vi "StopProcesses.vi"(8 "error in (no error)":errorcluster, 9 "timeout in ms (-1)":i32=-1, 11 "SMO":refnum<class "SMO.lvclass">) -> (0 "error out":errorcluster, 3 "SMO out":refnum<class "SMO.lvclass">)   [LabVIEW 2021, in "smo.lvlib" / "SMO.lvclass"]
doc: "Stops all processes in the JKI SMO.\n\n---------------------------------------------------------------\nJKI State Machine Objects™\nhttp://jki.net/state-machine-objects/\nCopyright (C) 2005-2015, JKI <info@jki.net>\nALL RIGHTS RESERVED"
uses:
  SMO.lvclass
  Typedefs/SMOState --Enum.ctl
  SMO.lvclass/SMO.ctl
  Protected/GetProtectedEvents.vi
  ReftoDVR--SMO.vi
panel:
  # "For instructions on how to use the JKI State Machine Objects, examples and video tutorials, visit:\nhttp://jki.net/state-machine-objects/\n\nJKI State Machine Objects™\nhttp://jki.net/state-machine-objects/\nCopyright (C) 2005-2015, JKI <info@jki.net>\nALL RIGHTS RESERVED"
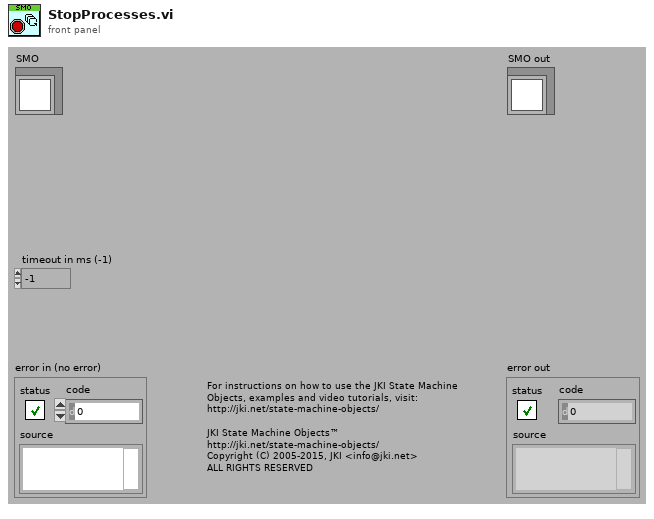
[diagram p1: front panel]
types:
  T1 = typedef "smo.lvlib/SMO.lvclass/SMOState --Enum.ctl" = enum16{"unknown", "Created", "Started", "Stopped"}
  T2 = typedef "smo.lvlib/SMO.lvclass/Process Error Notification--Cluster.ctl" = cluster{"error":errorcluster}
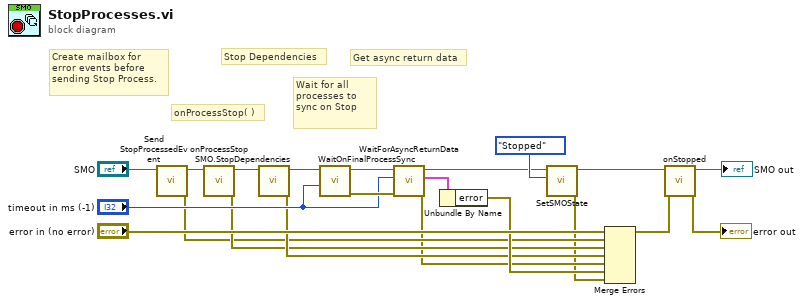
[diagram p0: block diagram]
diagram:
  # "Stop Dependencies"
  # "Get async return data"
  # "Wait for all processes to sync on Stop"
  # "onProcessStop( )"
  # "Create mailbox for\nerror events before\nsending Stop Process."
  n1 = call "Send StopProcessedEvent.vi"("SMO"="SMO") -> ("error out"=w7:errorcluster, "SMO out"=w20:refnum<class "SMO.lvclass">)  [unwired: 9 in]
  n2 = call-dynamic "onProcessStop.vi"("SMO"=w20) -> ("error out"=w8:errorcluster, "SMO out"=w12:refnum<class "SMO.lvclass">)  [unwired: 9 in]
  n3 = call "SMO.StopDependencies.vi"("SMO in"=w12) -> ("error out"=w9:errorcluster, "SMO out"=w11:refnum<class "SMO.lvclass">)  [unwired: 9 in]
  n4 = call "WaitOnFinalProcessSync.vi"("timeout in ms (-1)"="timeout in ms (-1)", "SMO"=w11) -> ("error out"=w14:errorcluster, "SMO out"=w15:refnum<class "SMO.lvclass">)  [unwired: 8 in]
  n5 = call "WaitForAsyncReturnData.vi"("error in (no error)"=w14, "timeout in ms (-1)"="timeout in ms (-1)", "SMO"=w15) -> ("error out"=w6:errorcluster, "Process Notification"=w16:T2, "SMO out"=w5:refnum<class "SMO.lvclass">)  [unwired: 6 in]
  n6 = Unbundle By Name(w16) -> ("error"=w10:errorcluster)
  n7 = call "SetSMOState.vi"("SMO State"=SMOState_--Enum."Stopped" ("event data"), "SMO in"=w5) -> ("error out"=w3:errorcluster, "SMO out"=w4:refnum<class "SMO.lvclass">)  [unwired: 8 in]
  n8 = Merge Errors("error in (no error)", w7, w8, w9, w6, w10, w3) -> (w2:errorcluster)
  n9 = call-dynamic "onStopped.vi"("error in (no error)"=w2, "SMO"=w4) -> ("error out"=→"error out":errorcluster, "SMO out"=→"SMO out":refnum<class "SMO.lvclass">)  [unwired: 8 in]
